vi "数据回放.vi"() -> ()   [LabVIEW 2012]
uses:
  <vilib>/Utility/file.llb/Read From Spreadsheet File (DBL).vi
  <vilib>/Analysis/NI_AALPro.lvlib
  <vilib>/Analysis/4window.llb/Hanning Window (DBL).vi
  <vilib>/Analysis/2dsp.llb/Real FFT.vi
  <vilib>/Analysis/4window.llb/Hamming Window (DBL).vi
  <vilib>/Analysis/4window.llb/Blackman Window (DBL).vi
  <vilib>/Analysis/NI_AALBase.lvlib
  <vilib>/Analysis/3filter.llb/Butterworth Filter (DBL).vi
  <vilib>/Analysis/3filter.llb/Filter Passband Type.ctl
panel:
  in  "filter type":T1 caption="滤波器类型"
  in  "?":u16(ring) items=["hanning", "hamming", "blackman"]
  in  "退出":bool
  in  "重置":bool
  out "波形图表 3":dbl[][](graph)
  out "波形图表 2":dbl[][](graph)
  out "波形图表":dbl[][](graph)
  # "数据回放"
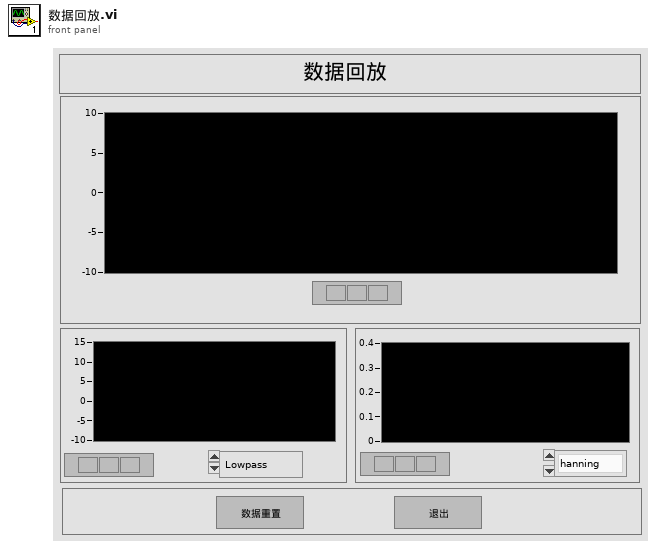
[diagram p1: front panel]
types:
  T1 = typedef "NI_AALBase.lvlib/Filter Passband Type.ctl" = enum32{"Lowpass", "Highpass", "Bandpass", "Bandstop"}
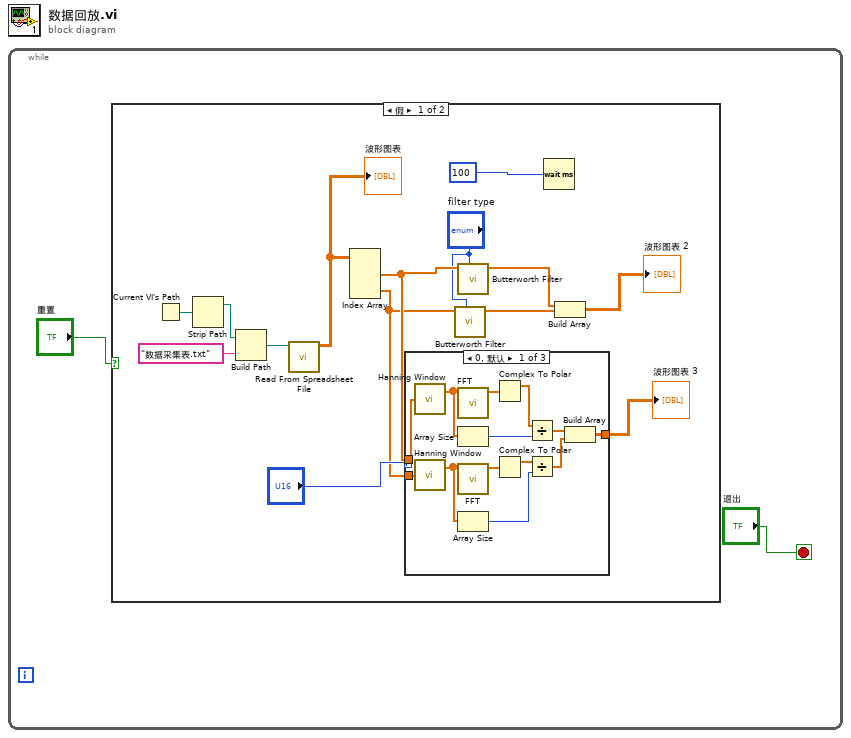
[diagram p0: block diagram]
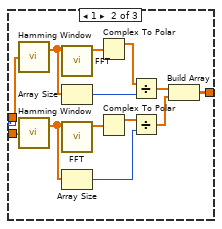
[diagram p2: hidden frame]
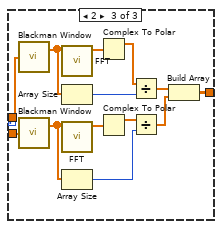
[diagram p3: hidden frame]
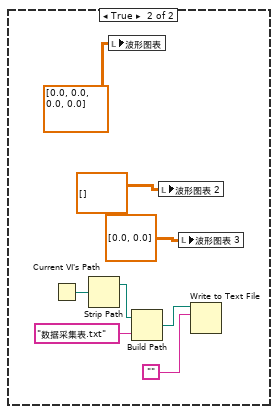
[diagram p4: hidden frame]
diagram:
  n1 = while {
    stop <- "退出" stop-if-true
    n2 = case shown="假" "重置" {
      frame False {
        n3 = Current VI's Path() -> (path=w14:path)
        n4 = Strip Path(path=w14) -> (stripped path=w15:path)  [unwired: 1 out]
        n5 = Build Path(base path=w15, name or relative path="数据采集表.txt") -> (appended path=w16:path)
        n6 = call-poly <vilib>:"Read From Spreadsheet File.vi"("file path (dialog if empty)"=w16) -> ("all rows"=w9:dbl[][])  [unwired: 6 in, 4 out]
        "波形图表" <- w9
        n7 = Index Array(array=w9) -> (element #1=w8:dbl[], element #2=w6:dbl[])  [unwired: 4 in]
        n8 = case shown="0, 默认" "?" {
          tunnel: w8 -> [w29 w42 w55]
          tunnel: w6 -> [w28 w41 w54]
          tunnel: [w27 w40 w53] -> w11
          frame 0, Default {
            n9 = call-poly <vilib>:"Hanning Window.vi"("X"=w29) -> ("Windowed X"=w17:dbl[])  [unwired: 1 out]
            n10 = call-poly <vilib>:"Hanning Window.vi"("X"=w28) -> ("Windowed X"=w25:dbl[])  [unwired: 1 out]
            n11 = call-poly <vilib>:"FFT.vi"("X"=w17) -> ("FFT {X}"=w19:cdb[])  [unwired: 9 in, 1 out]
            n12 = Array Size(array=w17) -> (size(s)=w21:i32)
            n13 = call-poly <vilib>:"FFT.vi"("X"=w25) -> ("FFT {X}"=w26:cdb[])  [unwired: 9 in, 1 out]
            n14 = Array Size(array=w25) -> (size(s)=w23:i32)
            n15 = Complex To Polar(r * e^(i*theta)=w19) -> (r=w20:dbl[])  [unwired: 1 out]
            n16 = Complex To Polar(r * e^(i*theta)=w26) -> (r=w24:dbl[])  [unwired: 1 out]
            n17 = Divide(x=w20, y=w21) -> (x/y=w18:dbl[])
            n18 = Divide(x=w24, y=w23) -> (x/y=w22:dbl[])
            n19 = Build Array(w18, w22) -> (w27:dbl[][])
          }
          frame 1 {
            n20 = call-poly <vilib>:"Hamming Window.vi"("X"=w42) -> ("Windowed X"=w30:dbl[])  [unwired: 1 out]
            n21 = call-poly <vilib>:"Hamming Window.vi"("X"=w41) -> ("Windowed X"=w38:dbl[])  [unwired: 1 out]
            n22 = call-poly <vilib>:"FFT.vi"("X"=w30) -> ("FFT {X}"=w32:cdb[])  [unwired: 9 in, 1 out]
            n23 = Array Size(array=w30) -> (size(s)=w34:i32)
            n24 = call-poly <vilib>:"FFT.vi"("X"=w38) -> ("FFT {X}"=w39:cdb[])  [unwired: 9 in, 1 out]
            n25 = Array Size(array=w38) -> (size(s)=w36:i32)
            n26 = Complex To Polar(r * e^(i*theta)=w32) -> (r=w33:dbl[])  [unwired: 1 out]
            n27 = Complex To Polar(r * e^(i*theta)=w39) -> (r=w37:dbl[])  [unwired: 1 out]
            n28 = Divide(x=w33, y=w34) -> (x/y=w31:dbl[])
            n29 = Divide(x=w37, y=w36) -> (x/y=w35:dbl[])
            n30 = Build Array(w31, w35) -> (w40:dbl[][])
          }
          frame 2 {
            n31 = call-poly <vilib>:"Blackman Window.vi"("X"=w55) -> ("Windowed X"=w43:dbl[])  [unwired: 1 out]
            n32 = call-poly <vilib>:"Blackman Window.vi"("X"=w54) -> ("Windowed X"=w51:dbl[])  [unwired: 1 out]
            n33 = call-poly <vilib>:"FFT.vi"("X"=w43) -> ("FFT {X}"=w45:cdb[])  [unwired: 9 in, 1 out]
            n34 = Array Size(array=w43) -> (size(s)=w47:i32)
            n35 = call-poly <vilib>:"FFT.vi"("X"=w51) -> ("FFT {X}"=w52:cdb[])  [unwired: 9 in, 1 out]
            n36 = Array Size(array=w51) -> (size(s)=w49:i32)
            n37 = Complex To Polar(r * e^(i*theta)=w45) -> (r=w46:dbl[])  [unwired: 1 out]
            n38 = Complex To Polar(r * e^(i*theta)=w52) -> (r=w50:dbl[])  [unwired: 1 out]
            n39 = Divide(x=w46, y=w47) -> (x/y=w44:dbl[])
            n40 = Divide(x=w50, y=w49) -> (x/y=w48:dbl[])
            n41 = Build Array(w44, w48) -> (w53:dbl[][])
          }
        }
        "波形图表 3" <- w11
        n42 = call-poly <vilib>:"Butterworth Filter.vi"("filter type"="filter type", "X"=w6) -> ("Filtered X"=w5:dbl[])  [unwired: 6 in, 1 out]
        n43 = call-poly <vilib>:"Butterworth Filter.vi"("filter type"="filter type", "X"=w8) -> ("Filtered X"=w7:dbl[])  [unwired: 6 in, 1 out]
        n44 = Wait (ms)(milliseconds to wait=u32 100 ("等待时间（毫秒）")) -> ()  [unwired: 1 out]
        n45 = Build Array(w7, w5) -> (→"波形图表 2":dbl[][])
      }
      frame True {
        n46 = Current VI's Path() -> (path=w62:path)
        n47 = Strip Path(path=w62) -> (stripped path=w61:path)  [unwired: 1 out]
        n48 = local write "波形图表"(dbl[][] [[0.0, 0.0], [0.0, 0.0]] ("all rows")) -> ()
        n49 = Build Path(base path=w61, name or relative path="数据采集表.txt") -> (appended path=w59:path)
        n50 = local write "波形图表 2"(dbl[][] [] ("波形图表 2")) -> ()
        n51 = local write "波形图表 3"(dbl[][] [[0.0], [0.0]] ("波形图表 3")) -> ()
        n52 = Write to Text File(file (use dialog)=w59, text="") -> ()  [unwired: 2 in, 3 out]
      }
    }
  }
